vi "ReferencePath.vi"() -> (3 "relative path":path)   [LabVIEW 2009]
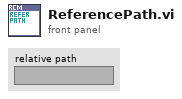
[diagram p1: front panel]
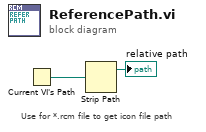
[diagram p0: block diagram]
diagram:
  # "Use for *.rcm file to get icon file path"
  n1 = Current VI's Path() -> (path=w2:path)
  n2 = Strip Path(path=w2) -> (stripped path=→"relative path":path)  [unwired: 1 out]
